vi "TestCloneAPI.vi"() -> ()   [LabVIEW 2014, in "FlagImpairModule.lvlib"]
uses:
  FlagImpairModule.lvlib
  PublicAPI/Arguments/Requests/clFlagImpairConfig.ctl
  PublicAPI/Arguments/Requests/dblFlagImpairParams.ctl
  PublicAPI/Arguments/Requests/dblTimeArray.ctl
  PublicAPI/Arguments/Broadcasts/ui32FlagImpairmentArray.ctl
  <userlib>/NIST/ModuleAdminLib/ModuleAdmin/ModuleAdmin.lvclass
  PublicAPI/Arguments/Broadcasts/clDidInit.ctl
  <userlib>/NIST/ModuleAdminLib/ModuleAdmin/ModuleAdmin.lvclass/ModuleAdmin.ctl
  PublicAPI/Arguments/Requests/clStopArgument.ctl
  PublicAPI/Arguments/Broadcasts/clStatUpdate.ctl
  PublicAPI/Arguments/Broadcasts/clErrorRpt.ctl
  <userlib>/NIST/ModuleAdminLib/ModuleAdmin/Accessors/Read CloneRegRef.vi
  <vilib>/Analysis/1siggen.llb/Ramp Pattern by Delta.vi
  <userlib>/NIST/ModuleAdminLib/CloneRegistration/CloneRegistration.lvclass
  <vilib>/Analysis/NI_AALBase.lvlib
panel:
  in  "Show Panel":bool=TRUE
  in  "btnGetFlags":bool
  out "ui32FlagImpairmentArray":T1
  out "dblTimeArray":T2
  in  "btnReadTimeArray":bool
  in  "btnWriteTimeArray":bool
  in  "ReportingRate":dbl=60.0
  in  "EndTime":dbl=1.0
  in  "StartTime":dbl
  in  "btnReadFlagImpairParams":bool
  out "dblFlagImpairParams Report":T3
  in  "btnWriteFlagImpairParams":bool
  in  "dblFlagImpairParams":T3=[[0.05], [0.5], [1.049e-10], [-6.709e-16], [2.73e-16]]
  in  "btnReadFlagImpairConfig":bool
  in  "btnWriteFlagImpairConfig":bool
  out "clFlagImpairConfig Report":T4 {"FlagImpairmentType" items=["Test0", "Test1"]}
  in  "clFlagImpairConfig":T4 {"FlagImpairmentType" items=["Test0", "Test1"]}
  in  "btnReadPluginPath":bool
  out "FlagImpairPluginINIFilePath Report":path
  in  "btnLoadPlugin":bool
  in  "FlagImpairPluginINIFilePath":path=path "P:/Framework/FlagImpairment/FlagImpairPlugins/C37.118FlagImpairPlugin/C37.118FlagImpairPlugin.ini"
  in  "btnRemove":bool
  out "Status Log":string
  out "Active Modules (Array)":string[](array[string])
  in  "btnAdd":bool
  in  "btnStop":bool
  in  "Select Module":i32(ring)=-1 caption="Select Module to send Request" items=["All"=-1, "4140002"=4140002, "4140003"=4140003]
  # "Hidden"
  # "Visible"
  # "The impairment \ntype is just a\nplaceholder for now."
  # "The impairment \ntype is just a\nplaceholder for now."
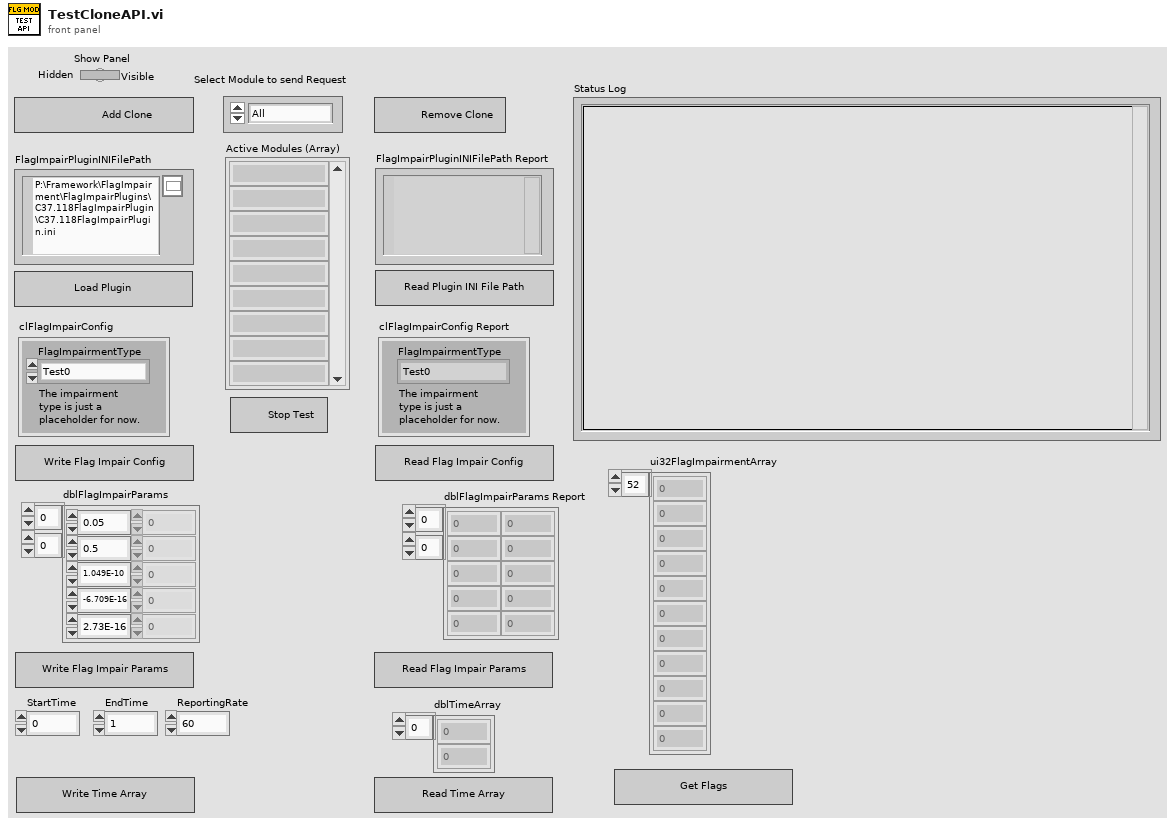
[diagram p1: front panel]
types:
  T1 = typedef "FlagImpairModule.lvlib/ui32FlagImpairmentArray.ctl" = u32[]
  T2 = typedef "FlagImpairModule.lvlib/dblTimeArray.ctl" = dbl[]
  T3 = typedef "FlagImpairModule.lvlib/dblFlagImpairParams.ctl" = dbl[][]
  T4 = typedef "FlagImpairModule.lvlib/clFlagImpairConfig.ctl" = cluster{"FlagImpairmentType":u16}
  T5 = typedef "FlagImpairModule.lvlib/clBroadcastEvents.ctl" = cluster{"DidInit":refnum<user-event>, "StatusUpdate":refnum<user-event>, "ErrorReport":refnum<user-event>, "DidStop":refnum<user-event>, "ReadFlagImpairConfig":refnum<user-event>, "ReadPluginINIFilePath":refnum<user-event>, "ReadFlagImpairParams":refnum<user-event>, "ReadTimeArray":refnum<user-event>, "GetFlagImpairment":refnum<user-event>}
  T6 = typedef "FlagImpairModule.lvlib/clDidInit.ctl" = cluster{"Init?":bool, "ModuleAdmin":refnum<class "ModuleAdmin.lvclass">}
  T7 = typedef "FlagImpairModule.lvlib/clStopArgument.ctl" = cluster{"Exit via Stop Module Req?":bool, "Wait for Module to stop?":bool, "ModuleAdmin":refnum<class "ModuleAdmin.lvclass">}
  T8 = typedef "FlagImpairModule.lvlib/clStatUpdate.ctl" = cluster{"Status":string}
  T9 = typedef "FlagImpairModule.lvlib/clErrorRpt.ctl" = cluster{"error":errorcluster, "AdditionalInfo":string}
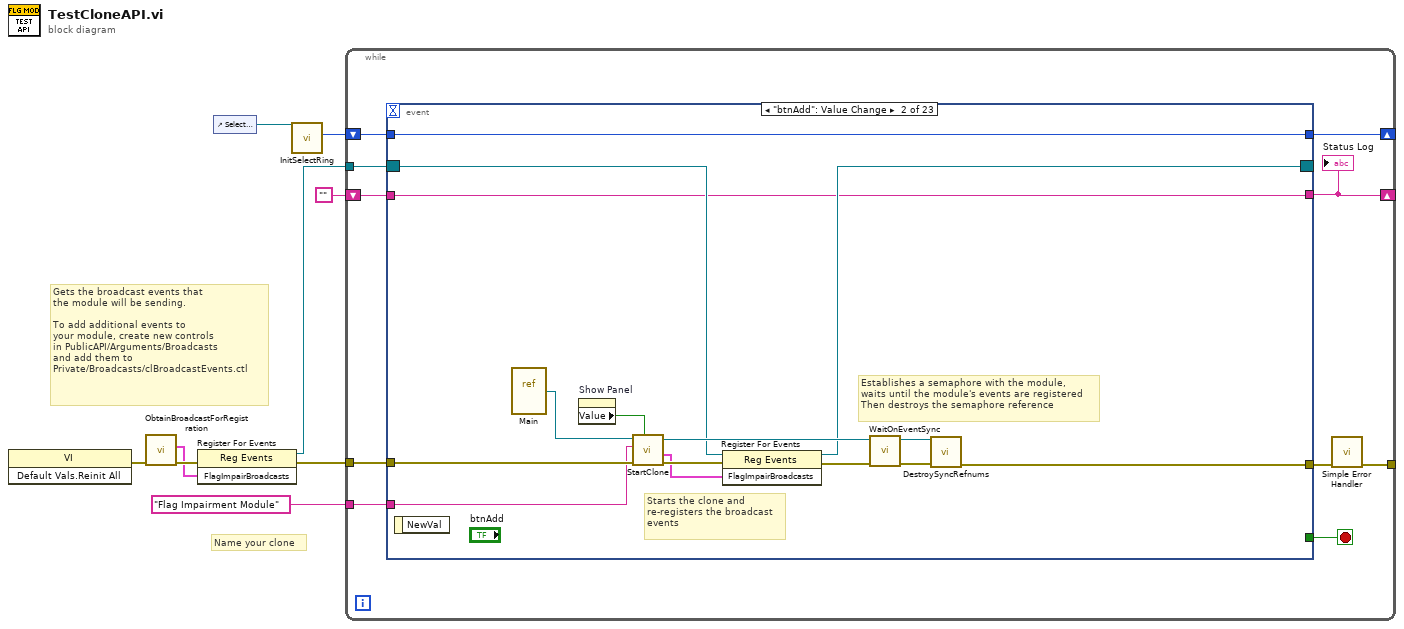
[diagram p0: block diagram]
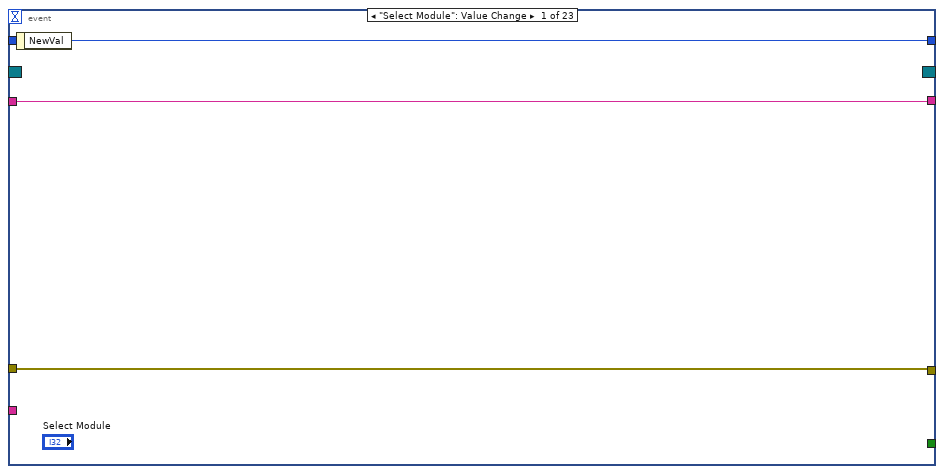
[diagram p2: hidden frame]
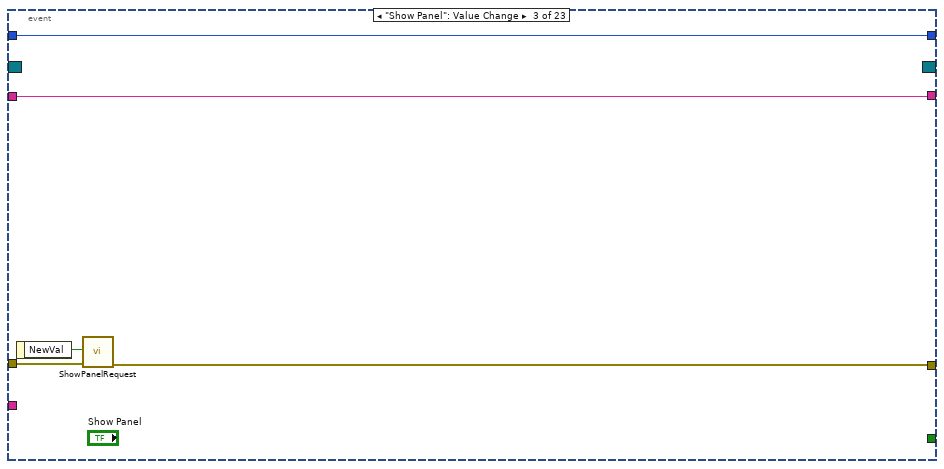
[diagram p3: hidden frame]
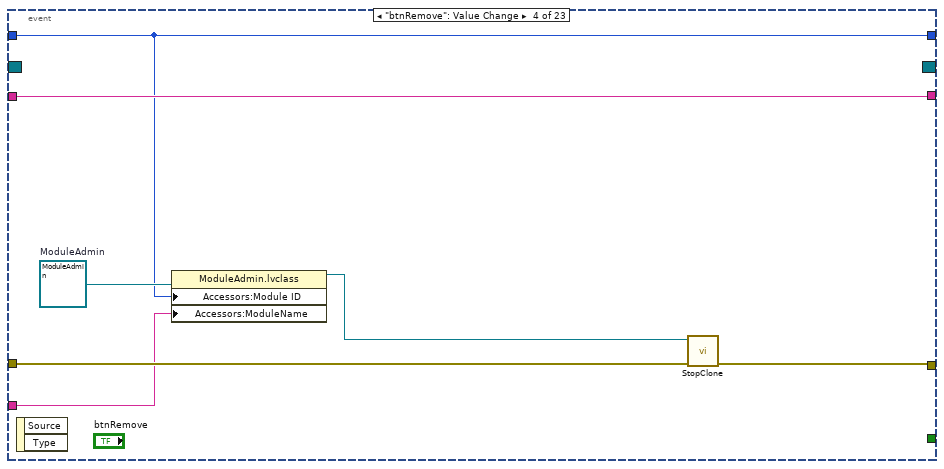
[diagram p4: hidden frame]
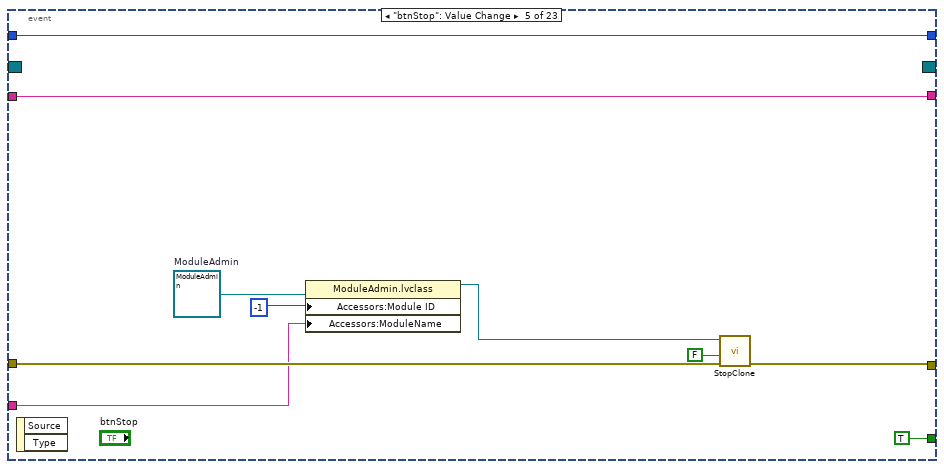
[diagram p5: hidden frame]
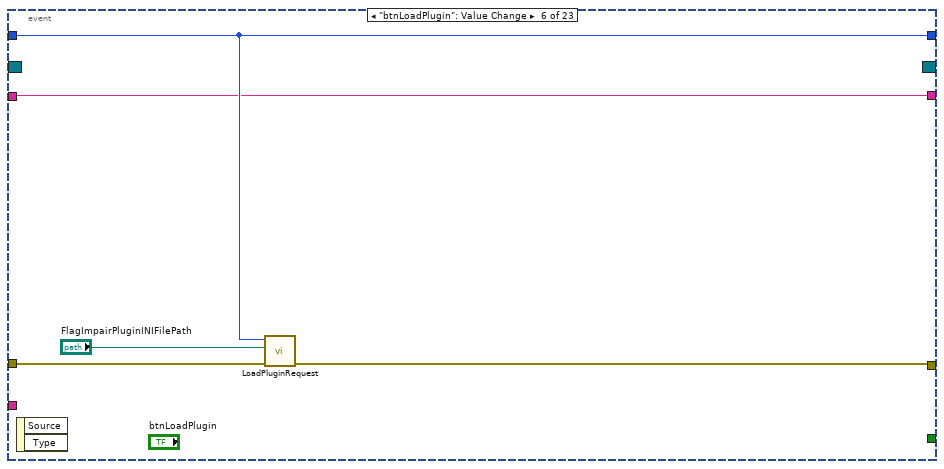
[diagram p6: hidden frame]
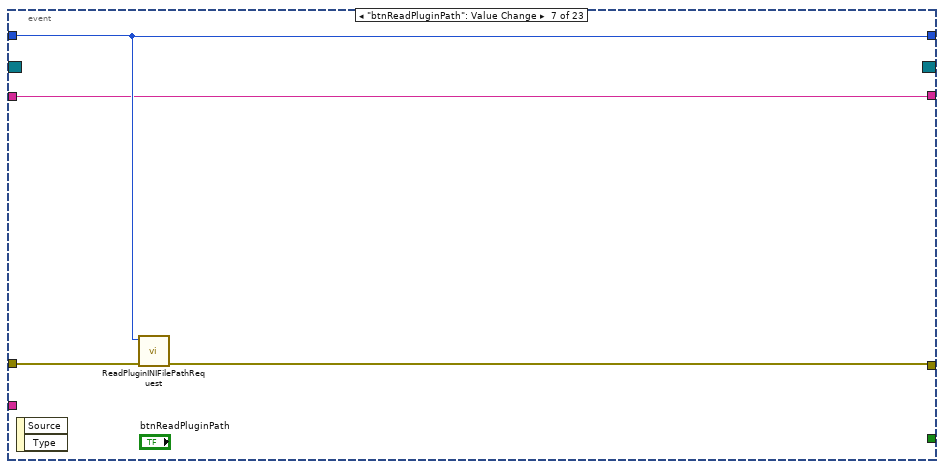
[diagram p7: hidden frame]
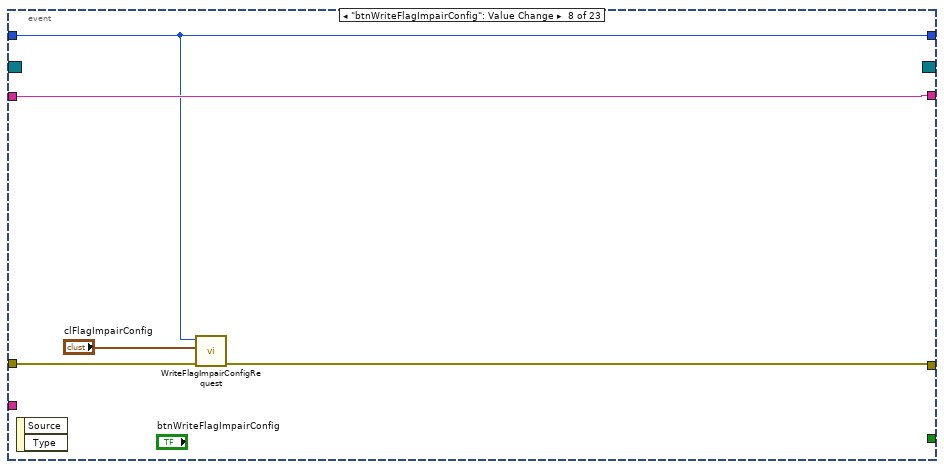
[diagram p8: hidden frame]
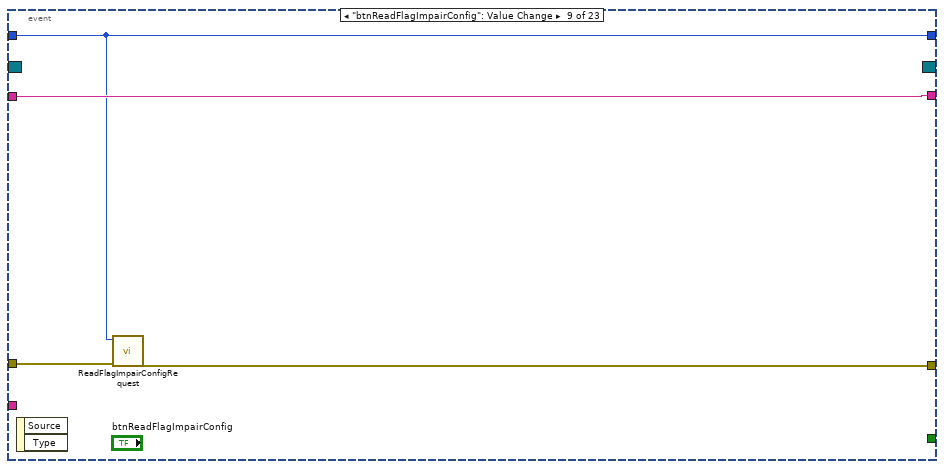
[diagram p9: hidden frame]
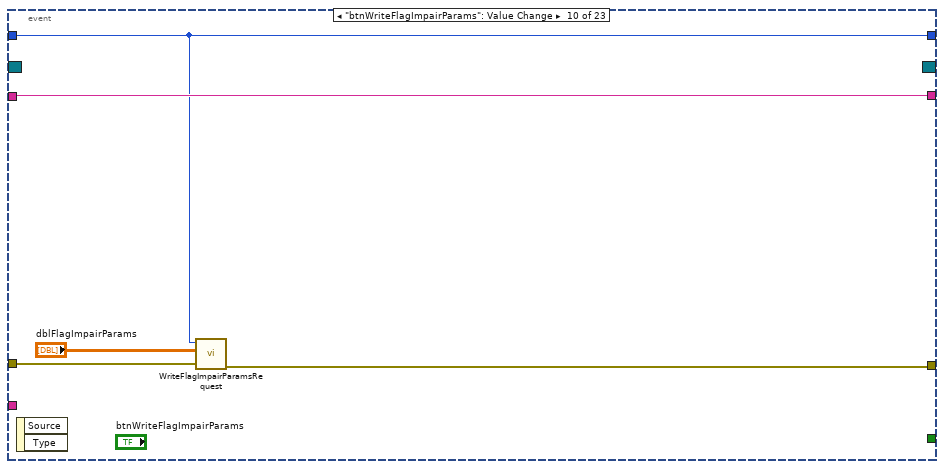
[diagram p10: hidden frame]
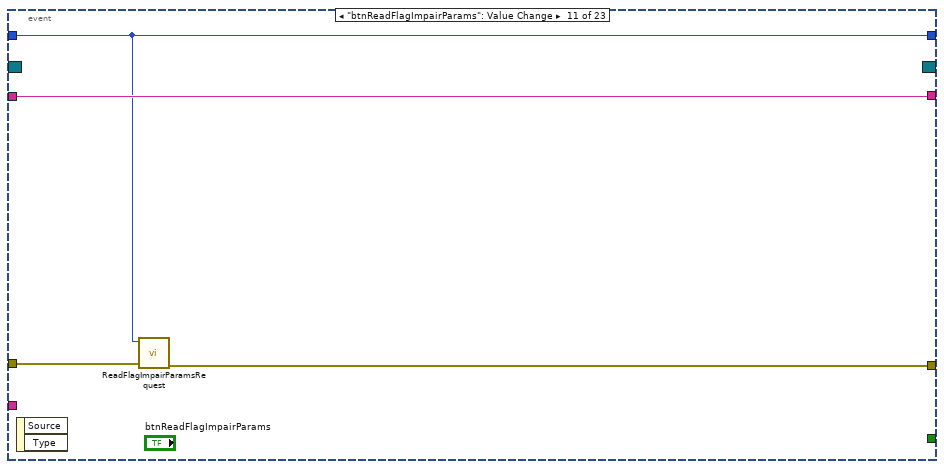
[diagram p11: hidden frame]
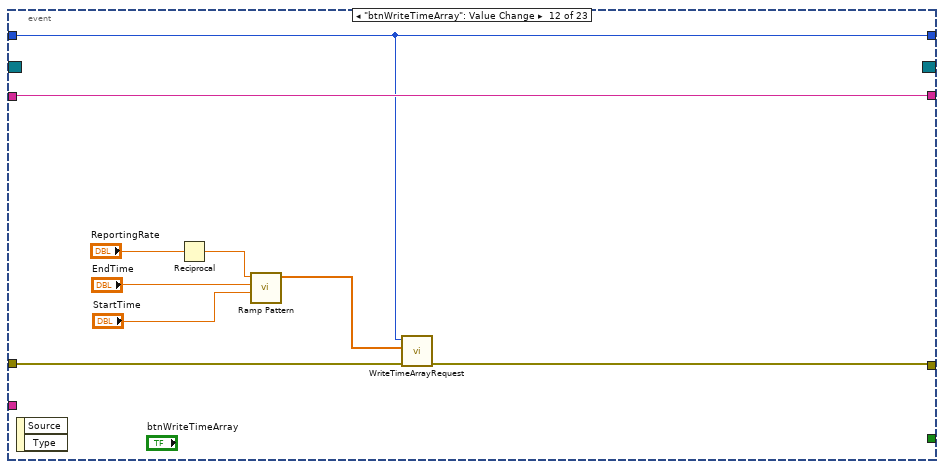
[diagram p12: hidden frame]
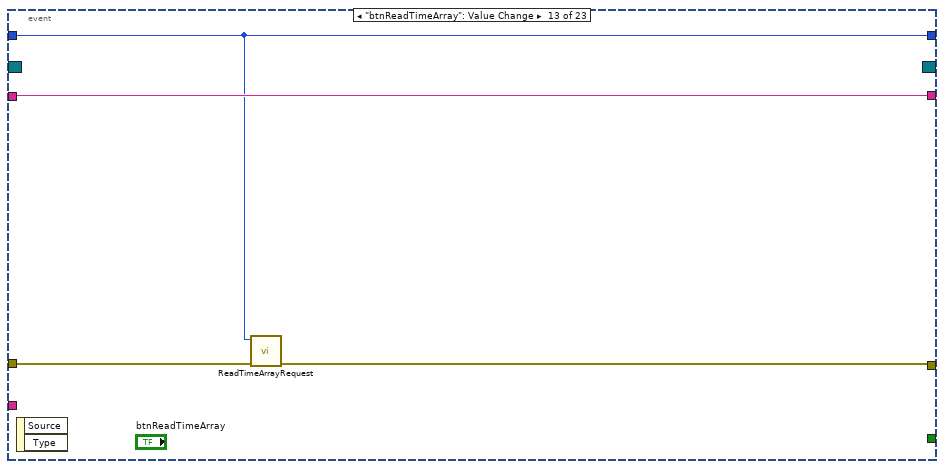
[diagram p13: hidden frame]
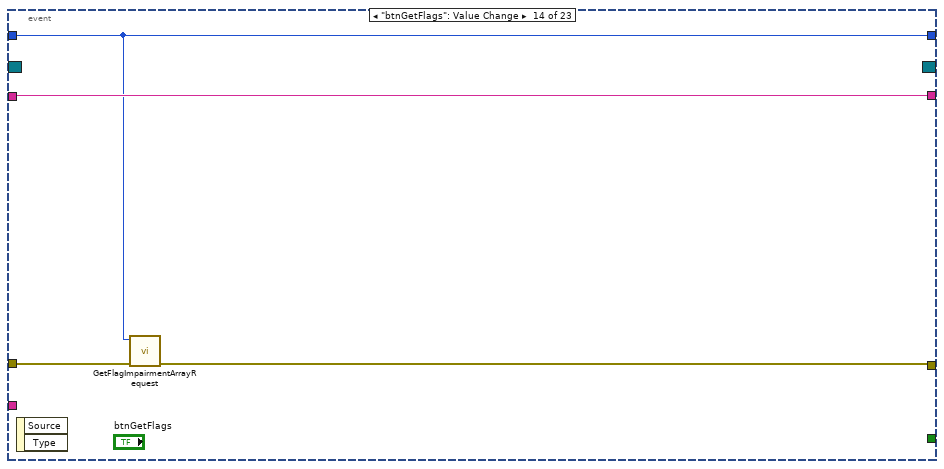
[diagram p14: hidden frame]
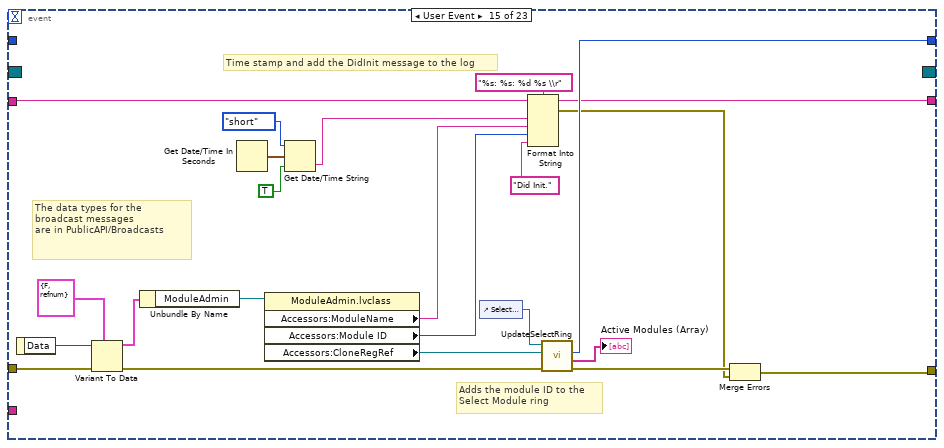
[diagram p15: hidden frame]
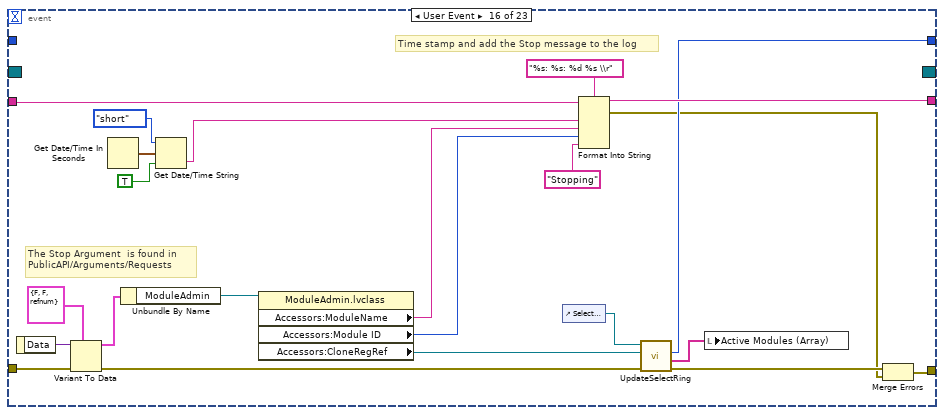
[diagram p16: hidden frame]
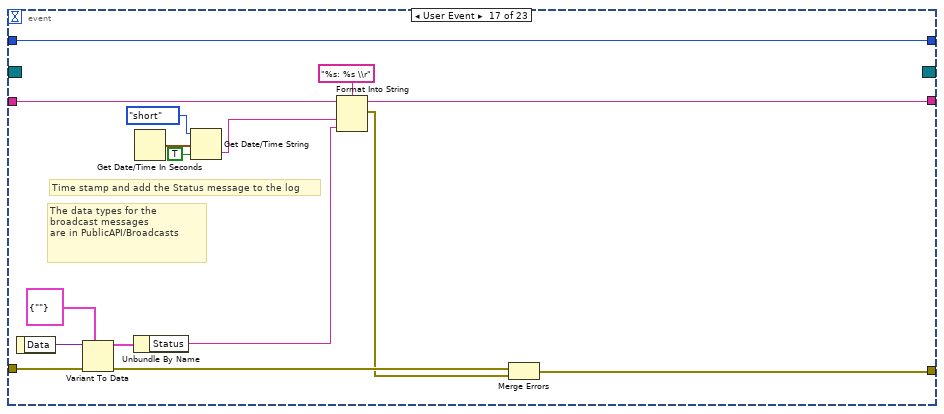
[diagram p17: hidden frame]
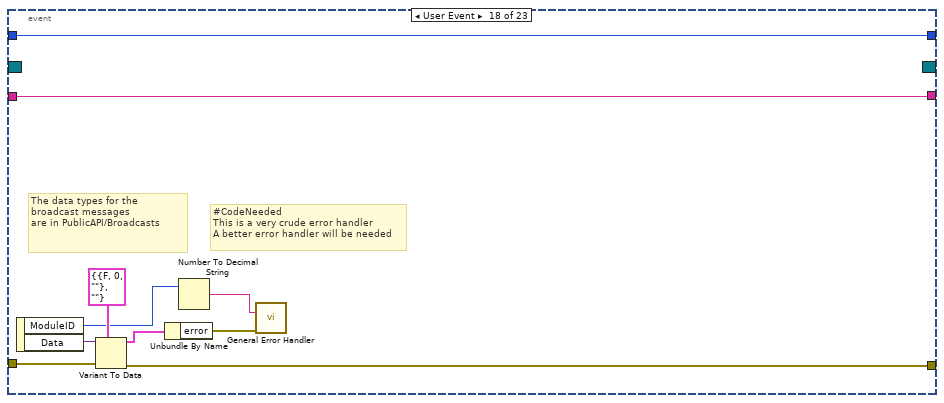
[diagram p18: hidden frame]
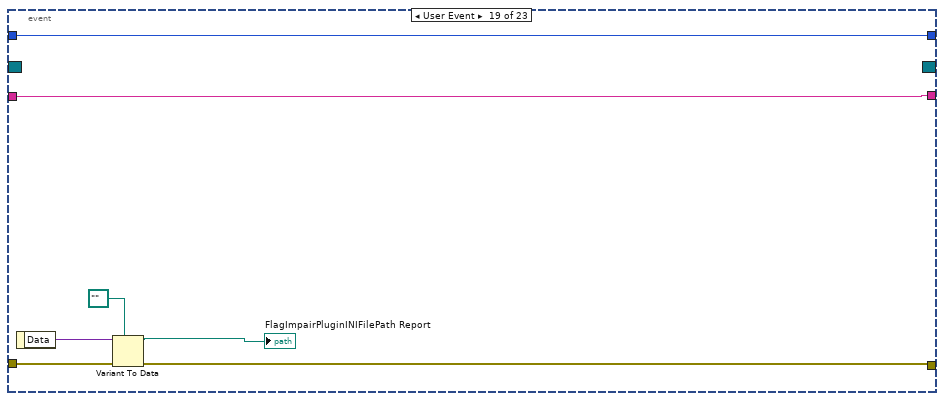
[diagram p19: hidden frame]
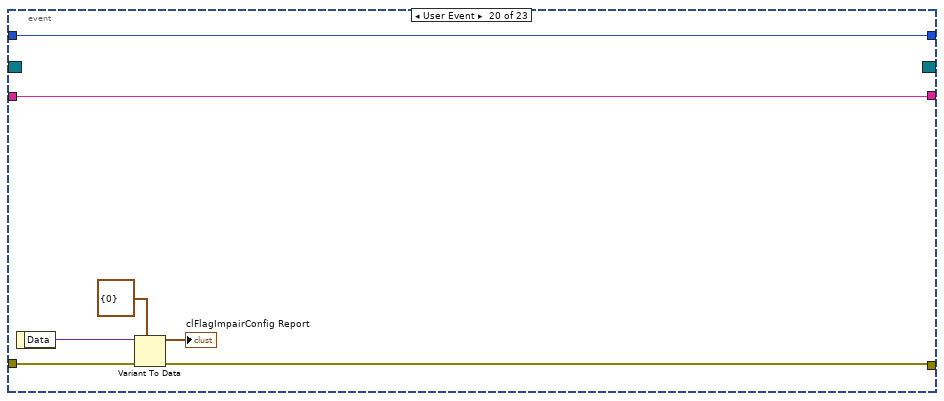
[diagram p20: hidden frame]
diagram:
  # "Name your clone"
  # "Gets the broadcast events that\nthe module will be sending.\n\nTo add additional events to\nyour module, create new controls\nin PublicAPI/Arguments/Broadcasts\nand add them to\nPrivate/Broadcasts/clBroadcastEvents.ctl"
  n1 = invoke class="VI" method="Default Vals.Reinit All"() -> (error out=w7:errorcluster)  [unwired: 3 in, 2 out]
  n2 = call "ObtainBroadcastForRegistration.vi"("error in (no error)"=w7) -> ("error out"=w6:errorcluster, "FlagImpairBroadcasts"=w5:T5)  [unwired: 9 in]
  n3 = register-events(error in=w6, w5) -> (reference out=w3:refnum<event-registration>, error out=w4:errorcluster)  [unwired: 1 in]
  n4 = control-ref of="Select Module"() -> (w9:refnum<vi>)
  n5 = call "InitSelectRing.vi"("Ring Refnum"=w9) -> ("Module Ring Value"=w8:i32)  [unwired: 9 in, 1 out]
  n6 = while {
    shift-right: [w18] -> _
    shift-left: w8 -> [w19]
    tunnel: w4 -> [w16]
    tunnel: w3 -> [w13]
    tunnel: [w14] -> _
    shift-right: [w12] -> _
    shift-left: "" -> [w11]
    tunnel: "Flag Impairment Module" ("ModuleName") -> [w10]
    stop <- w17 stop-if-true
    n7 = event shown="[1] \"btnAdd\": Value Change" {
      selector: w13 -> [_ w28 _ _ _ _ _ _ _ _ _ _ _ _ _ _ _ _ _ _ _ _ _]
      dyn-events: [_ w27 _ _ _ _ _ _ _ _ _ _ _ _ _ _ _ _ _ _ _ _ _] -> _
      timeout: _ -> [_ _ _ _ _ _ _ _ _ _ _ _ _ _ _ _ _ _ _ _ _ _ _]
      tunnel: w19 -> [_ w37 w38 w45 w59 w62 w67 w70 w74 w79 w83 w89 w96 w101 _ _ w165 w167 w177 w184 w191 w197 w206]
      tunnel: [w22 w37 w38 w45 w59 w62 w67 w70 w74 w79 w83 w89 w96 w101 w121 w136 w165 w167 w177 w184 w191 w197 w206] -> w18
      tunnel: [_ _ _ _ TRUE _ _ _ _ _ _ _ _ _ _ _ _ _ _ _ _ _ _] -> w17
      tunnel: w16 -> [w20 w36 w42 w48 w57 w64 w68 w73 w77 w82 w86 w91 w98 w102 w126 w145 w162 w174 w182 w188 w195 w202 w210]
      tunnel: [w20 w29 w40 w47 w55 w60 w65 w69 w76 w78 w85 w90 w97 w100 w110 w133 w153 w173 w179 w185 w194 w201 w207] -> w15
      tunnel: [w21 w25 w39 w49 w54 w61 w66 w71 w75 w80 w84 w92 w99 w103 w114 w142 w156 w166 w178 w183 w190 w198 w205] -> w12
      tunnel: w11 -> [w21 w25 w39 w49 w54 w61 w66 w71 w75 w80 w84 w92 w99 w103 w113 w143 w164 w166 w178 w183 w190 w198 w205]
      tunnel: w10 -> [_ w24 _ w44 w51 _ _ _ _ _ _ _ _ _ _ _ _ _ _ _ _ _ _]
      event "Select Module": Value Change {
        n8 = event-data() -> ("NewVal"=w22:i32)  [unwired: 1 in]
      }
      event "btnAdd": Value Change {
        # "Establishes a semaphore with the module,\nwaits until the module's events are registered\nThen destroys the semaphore reference"
        # "Starts the clone and\nre-registers the broadcast \nevents"
        n9 = event-data() -> ()  [unwired: 1 in, 1 out]
        n10 = vi-ref "Main.vi"() -> (w26:refnum<vi>)
        n11 = property on="Show Panel" class="Bool (strict)"() -> ("Value"=w23:bool)  [unwired: 2 in, 2 out]
        n12 = call "StartClone.vi"("ShowPanel?"=w23, "error in (no error)"=w36, "ModuleName"=w24, "VI Refnum"=w26) -> ("error out"=w35:errorcluster, "FlagImpairBroadcast"=w30:T5, "ModuleAdmin"=w32:refnum<class "ModuleAdmin.lvclass">)  [unwired: 5 in]
        n13 = register-events(reference=w28, error in=w35, w30) -> (reference out=w27:refnum<event-registration>, error out=w34:errorcluster)
        n14 = call <userlib>:"WaitOnEventSync.vi"("error in (no error)"=w34, "ModuleAdmin"=w32) -> ("error out"=w33:errorcluster, "ModuleAdmin"=w31:refnum<class "ModuleAdmin.lvclass">)  [unwired: 8 in]
        n15 = call <userlib>:"DestroySyncRefnums.vi"("error in (no error)"=w33, "ModuleAdmin"=w31) -> ("error out"=w29:errorcluster)  [unwired: 9 in]
      }
      event "Show Panel": Value Change {
        n16 = event-data() -> ("NewVal"=w41:bool)  [unwired: 1 in]
        n17 = call "ShowPanelRequest.vi"("error in (no error)"=w42, "ShowPanel?"=w41) -> ("error out"=w40:errorcluster)  [unwired: 9 in]
      }
      event "btnRemove": Value Change {
        w46 = refnum<class "ModuleAdmin.lvclass"> refnum  # ModuleAdmin
        n18 = event-data() -> ()  [unwired: 1 in, 2 out]
        n19 = property class="ModuleAdmin.lvclass"(reference=w46, "Accessors:Module ID"=w45, "Accessors:ModuleName"=w44) -> (reference out=w43:refnum<class "ModuleAdmin.lvclass">)  [unwired: 1 in, 1 out]
        n20 = call "StopClone.vi"("error in (no error)"=w48, "ModuleAdmin"=w43) -> ("error out"=w47:errorcluster)  [unwired: 9 in]
      }
      event "btnStop": Value Change {
        w53 = refnum<class "ModuleAdmin.lvclass"> refnum  # ModuleAdmin
        n21 = event-data() -> ()  [unwired: 1 in, 2 out]
        n22 = property class="ModuleAdmin.lvclass"(reference=w53, "Accessors:Module ID"=-1 ("Module ID"), "Accessors:ModuleName"=w51) -> (reference out=w50:refnum<class "ModuleAdmin.lvclass">)  [unwired: 1 in, 1 out]
        n23 = call "StopClone.vi"("error in (no error)"=w57, "Wait for Module to stop?"=FALSE, "ModuleAdmin"=w50) -> ("error out"=w55:errorcluster)  [unwired: 8 in]
      }
      event "btnLoadPlugin": Value Change {
        n24 = event-data() -> ()  [unwired: 1 in, 2 out]
        n25 = call "LoadPluginRequest.vi"("error in (no error)"=w64, "PathToPlugin"="FlagImpairPluginINIFilePath", "ModuleID"=w62) -> ("error out"=w60:errorcluster)  [unwired: 8 in]
      }
      event "btnReadPluginPath": Value Change {
        n26 = event-data() -> ()  [unwired: 1 in, 2 out]
        n27 = call "ReadPluginINIFilePathRequest.vi"("error in (no error)"=w68, "ModuleID"=w67) -> ("error out"=w65:errorcluster)  [unwired: 9 in]
      }
      event "btnWriteFlagImpairConfig": Value Change {
        n28 = event-data() -> ()  [unwired: 1 in, 2 out]
        n29 = call "WriteFlagImpairConfigRequest.vi"("error in (no error)"=w73, "clFlagImpairConfig"="clFlagImpairConfig", "ModuleID"=w70) -> ("error out"=w69:errorcluster)  [unwired: 8 in]
      }
      event "btnReadFlagImpairConfig": Value Change {
        n30 = event-data() -> ()  [unwired: 1 in, 2 out]
        n31 = call "ReadFlagImpairConfigRequest.vi"("error in (no error)"=w77, "ModuleID"=w74) -> ("error out"=w76:errorcluster)  [unwired: 9 in]
      }
      event "btnWriteFlagImpairParams": Value Change {
        n32 = event-data() -> ()  [unwired: 1 in, 2 out]
        n33 = call "WriteFlagImpairParamsRequest.vi"("error in (no error)"=w82, "dblFlagImpairParams"="dblFlagImpairParams", "ModuleID"=w79) -> ("error out"=w78:errorcluster)  [unwired: 8 in]
      }
      event "btnReadFlagImpairParams": Value Change {
        n34 = event-data() -> ()  [unwired: 1 in, 2 out]
        n35 = call "ReadFlagImpairParamsRequest.vi"("error in (no error)"=w86, "ModuleID"=w83) -> ("error out"=w85:errorcluster)  [unwired: 9 in]
      }
      event "btnWriteTimeArray": Value Change {
        n36 = event-data() -> ()  [unwired: 1 in, 2 out]
        n37 = Reciprocal(x="ReportingRate") -> (1/x=w87:dbl)
        n38 = call-poly <vilib>:"Ramp Pattern.vi"("start"="StartTime", "end"="EndTime", "delta"=w87) -> ("Ramp Pattern"=w88:dbl[])  [unwired: 6 in, 2 out]
        n39 = call "WriteTimeArrayRequest.vi"("error in (no error)"=w91, "dblTimeArray"=w88, "ModuleID"=w89) -> ("error out"=w90:errorcluster)  [unwired: 8 in]
      }
      event "btnReadTimeArray": Value Change {
        n40 = event-data() -> ()  [unwired: 1 in, 2 out]
        n41 = call "ReadTimeArrayRequest.vi"("error in (no error)"=w98, "ModuleID"=w96) -> ("error out"=w97:errorcluster)  [unwired: 9 in]
      }
      event "btnGetFlags": Value Change {
        n42 = event-data() -> ()  [unwired: 1 in, 2 out]
        n43 = call "GetFlagImpairmentArrayRequest.vi"("error in (no error)"=w102, "ModuleID"=w101) -> ("error out"=w100:errorcluster)  [unwired: 9 in]
      }
      event User Event {
        # "Adds the module ID to the \nSelect Module ring"
        # "Time stamp and add the DidInit message to the log"
        # "The data types for the broadcast messages\nare in PublicAPI/Broadcasts"
        n44 = event-data() -> ("Data"=w125:variant)  [unwired: 1 in]
        n45 = Variant To Data(error in=w126, type=T6 {"Init?"=FALSE, "ModuleAdmin"=refnum} ("clDidInit"), Variant=w125) -> (data=w118:T6, error out=w123:errorcluster)
        n46 = Unbundle By Name(w118) -> ("ModuleAdmin"=w107:refnum<class "ModuleAdmin.lvclass">)
        n47 = Get Date/Time In Seconds() -> (seconds since 1Jan1904=w116:timestamp)
        n48 = property class="ModuleAdmin.lvclass"(reference=w107) -> ("Accessors:ModuleName"=w105:string, "Accessors:Module ID"=w106:i32, "Accessors:CloneRegRef"=w104:refnum<data-value>)  [unwired: 1 in, 2 out]
        n49 = Get Date/Time String(date format (0)=enum16{"short", "long", "abbreviated"}."short", seconds (now)=w116, want seconds? (F)=TRUE) -> (time string=w119:string)  [unwired: 1 out]
        n50 = control-ref of="Select Module"() -> (w122:refnum<vi>)
        n51 = Format Into String(format string="%s: %s: %d %s \\r", initial string=w113, w119, w105, w106, "Did Init.") -> (resulting string=w114:string, error out=w111:errorcluster)  [unwired: 1 in]
        n52 = call "UpdateSelectRing.vi"("error in (no error)"=w123, "CloneRegRef"=w104, "Ring Refnum"=w122) -> ("error out"=w112:errorcluster, "ActiveModules"=→"Active Modules (Array)":string[], "Module Ring Value"=w121:i32)  [unwired: 6 in]
        n53 = Merge Errors(w112, w111) -> (w110:errorcluster)
      }
      event User Event {
        # "Time stamp and add the Stop message to the log"
        # "The Stop Argument  is found in\nPublicAPI/Arguments/Requests"
        n54 = event-data() -> ("Data"=w144:variant)  [unwired: 1 in]
        n55 = Variant To Data(error in=w145, type=T7 {"Exit via Stop Module Req?"=FALSE, "Wait for Module to stop?"=FALSE, "ModuleAdmin"=refnum} ("Stop Argument"), Variant=w144) -> (data=w140:T7, error out=w139:errorcluster)
        n56 = Get Date/Time In Seconds() -> (seconds since 1Jan1904=w147:timestamp)
        n57 = Unbundle By Name(w140) -> ("ModuleAdmin"=w129:refnum<class "ModuleAdmin.lvclass">)
        n58 = Get Date/Time String(date format (0)=enum16{"short", "long", "abbreviated"}."short", seconds (now)=w147, want seconds? (F)=TRUE) -> (time string=w149:string)  [unwired: 1 out]
        n59 = property class="ModuleAdmin.lvclass"(reference=w129) -> ("Accessors:ModuleName"=w128:string, "Accessors:Module ID"=w127:i32, "Accessors:CloneRegRef"=w130:refnum<data-value>)  [unwired: 1 in, 2 out]
        n60 = control-ref of="Select Module"() -> (w138:refnum<vi>)
        n61 = Format Into String(format string="%s: %s: %d %s \\r", initial string=w143, w149, w128, w127, "Stopping") -> (resulting string=w142:string, error out=w134:errorcluster)  [unwired: 1 in]
        n62 = call "UpdateSelectRing.vi"("error in (no error)"=w139, "CloneRegRef"=w130, "Ring Refnum"=w138) -> ("error out"=w135:errorcluster, "ActiveModules"=w137:string[], "Module Ring Value"=w136:i32)  [unwired: 6 in]
        n63 = local write "Active Modules (Array)"(w137) -> ()
        n64 = Merge Errors(w135, w134) -> (w133:errorcluster)
      }
      event User Event {
        # "Time stamp and add the Status message to the log"
        # "The data types for the broadcast messages\nare in PublicAPI/Broadcasts"
        n65 = event-data() -> ("Data"=w161:variant)  [unwired: 1 in]
        n66 = Variant To Data(error in=w162, type=T8 {"Status"=""} ("clStatUpdate"), Variant=w161) -> (data=w159:T8, error out=w155:errorcluster)
        n67 = Unbundle By Name(w159) -> ("Status"=w157:string)
        n68 = Get Date/Time In Seconds() -> (seconds since 1Jan1904=w158:timestamp)
        n69 = Get Date/Time String(date format (0)=enum16{"short", "long", "abbreviated"}."short", seconds (now)=w158, want seconds? (F)=TRUE) -> (time string=w150:string)  [unwired: 1 out]
        n70 = Format Into String(format string="%s: %s \\r", initial string=w164, w150, w157) -> (resulting string=w156:string, error out=w154:errorcluster)  [unwired: 1 in]
        n71 = Merge Errors(w155, w154) -> (w153:errorcluster)
      }
      event User Event {
        # "#CodeNeeded\nThis is a very crude error handler\nA better error handler will be needed"
        # "The data types for the broadcast messages\nare in PublicAPI/Broadcasts"
        n72 = event-data() -> ("ModuleID"=w170:i32, "Data"=w175:variant)  [unwired: 1 in]
        n73 = Variant To Data(error in=w174, type=T9 {"error"={"status"=FALSE, "code"=0, "source"=""}, "AdditionalInfo"=""} ("Cluster"), Variant=w175) -> (data=w171:T9, error out=w173:errorcluster)
        n74 = Unbundle By Name(w171) -> ("error"=w169:errorcluster)
        n75 = Number To Decimal String(number=w170) -> (decimal integer string=w168:string)  [unwired: 1 in]
        n76 = call <vilib>:"General Error Handler.vi"("[error source] (\" \")"=w168, "error in (no error)"=w169) -> ()  [unwired: 9 in, 5 out]
      }
      event User Event {
        n77 = event-data() -> ("Data"=w181:variant)  [unwired: 1 in]
        n78 = Variant To Data(error in=w182, type=path "", Variant=w181) -> (data=→"FlagImpairPluginINIFilePath Report":path, error out=w179:errorcluster)
      }
      event User Event {
        n79 = event-data() -> ("Data"=w187:variant)  [unwired: 1 in]
        n80 = Variant To Data(error in=w188, type=T4 {"FlagImpairmentType"=0} ("clFlagImpairConfig"), Variant=w187) -> (data=→"clFlagImpairConfig Report":T4, error out=w185:errorcluster)
      }
      event User Event {
        w193 = T3 []  # dblFlagImpairParams
        n81 = event-data() -> ("Data"=w196:variant)  [unwired: 1 in]
        n82 = Variant To Data(error in=w195, type=w193, Variant=w196) -> (data=→"dblFlagImpairParams Report":T3, error out=w194:errorcluster)
      }
      event User Event {
        w199 = T2 []  # dblTimeArray
        n83 = event-data() -> ("Data"=w203:variant)  [unwired: 1 in]
        n84 = Variant To Data(error in=w202, type=w199, Variant=w203) -> (data=→"dblTimeArray":T2, error out=w201:errorcluster)
      }
      event User Event {
        w204 = T1 []  # ui32FlagImpairmentArray
        n85 = event-data() -> ("Data"=w209:variant)  [unwired: 1 in]
        n86 = Variant To Data(error in=w210, type=w204, Variant=w209) -> (data=→"ui32FlagImpairmentArray":T1, error out=w207:errorcluster)
      }
    }
    "Status Log" <- w12
    n87 = call <vilib>:"Simple Error Handler.vi"("error in (no error)"=w15) -> ("error out"=w14:errorcluster)  [unwired: 4 in, 4 out]
  }
